vi "Micrometer Heading.vi"() -> ()   [LabVIEW 2024]
uses:
  Library/Class/Renishaw-XL80/Renishaw-XL80.lvclass
  Library/Class/Renishaw-XL80_EMU/Renishaw-XL80_EMU.lvclass
  <vilib>/Utility/file.llb/Write Delimited Spreadsheet (string).vi
panel:
  in  "Nominal":dbl[](array[numeric]) format="%.6f"
  in  "Delete RG":bool
  in  "Delete RB":bool
  out "Signal":dbl(slide) scale=0.0..31.0
  in  "sign_mode":bool
  out "ScanCode 2":i16
  in  "Add DUT":bool
  out "Zero Value":dbl format="%_8f"
  out "Mat Temp":dbl[](array[numeric]) caption="Mat Temp(°C)"
  out "Air Temp":dbl caption="Air Temp(°C)"
  in  "Reset":bool
  in  "Connect":bool
  in  "Zero":bool
  out "Serial Number":string caption="Laser Device ID"
  out "Connected":bool
  in  "Read RB":bool
  in  "R1":dbl[](array[numeric]) format="%.6f"
  in  "Clear RB":bool
  in  "Clear Result":bool
  in  "Export to CSV":bool
  in  "Calculate_Save":bool
  in  "Calculation Result":string[][](table)
  in  "Read RG":bool
  in  "R2":dbl[](array[numeric]) format="%.6f"
  in  "Clear RG":bool
  in  "Precision":u16(ring)=4 items=["0 digit", "1 digit", "2 digits", "3 digits", "4 digits", "5 digits", "6 digits"]
  in  "Unit":u16(ring) caption="mm/inch" items=["mm", "inch"]
  out "Measurement":dbl format="%.6f"
  in  "Description":string
  in  "Mat Exp Coef":dbl format="%_4f"
  in  "Manufacturer":string
  in  "Ref equipment ID":string
  in  "Model No.":string
  in  "S/No. or ID":string
  in  "Job No.":string
  out "uncalibrated":dbl
  out "error out 2":errorcluster
  out "ScanCode":i16
  out "mat_c":dbl
  out "C":dbl format="%.7f"
  out "error out":errorcluster
  in  "error IO":errorcluster
  # "Job Info"
  # "Test Parameters"
  # "DUT Info"
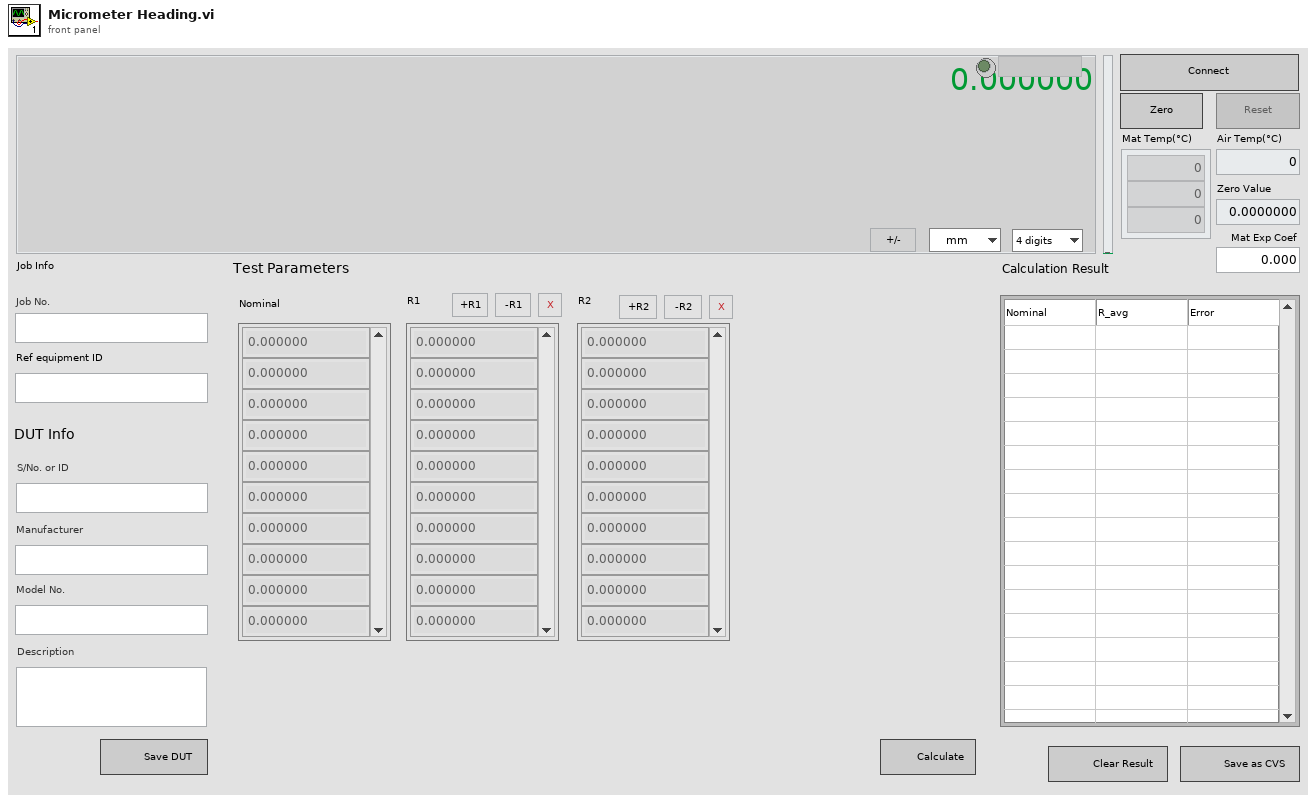
[diagram p1: front panel]
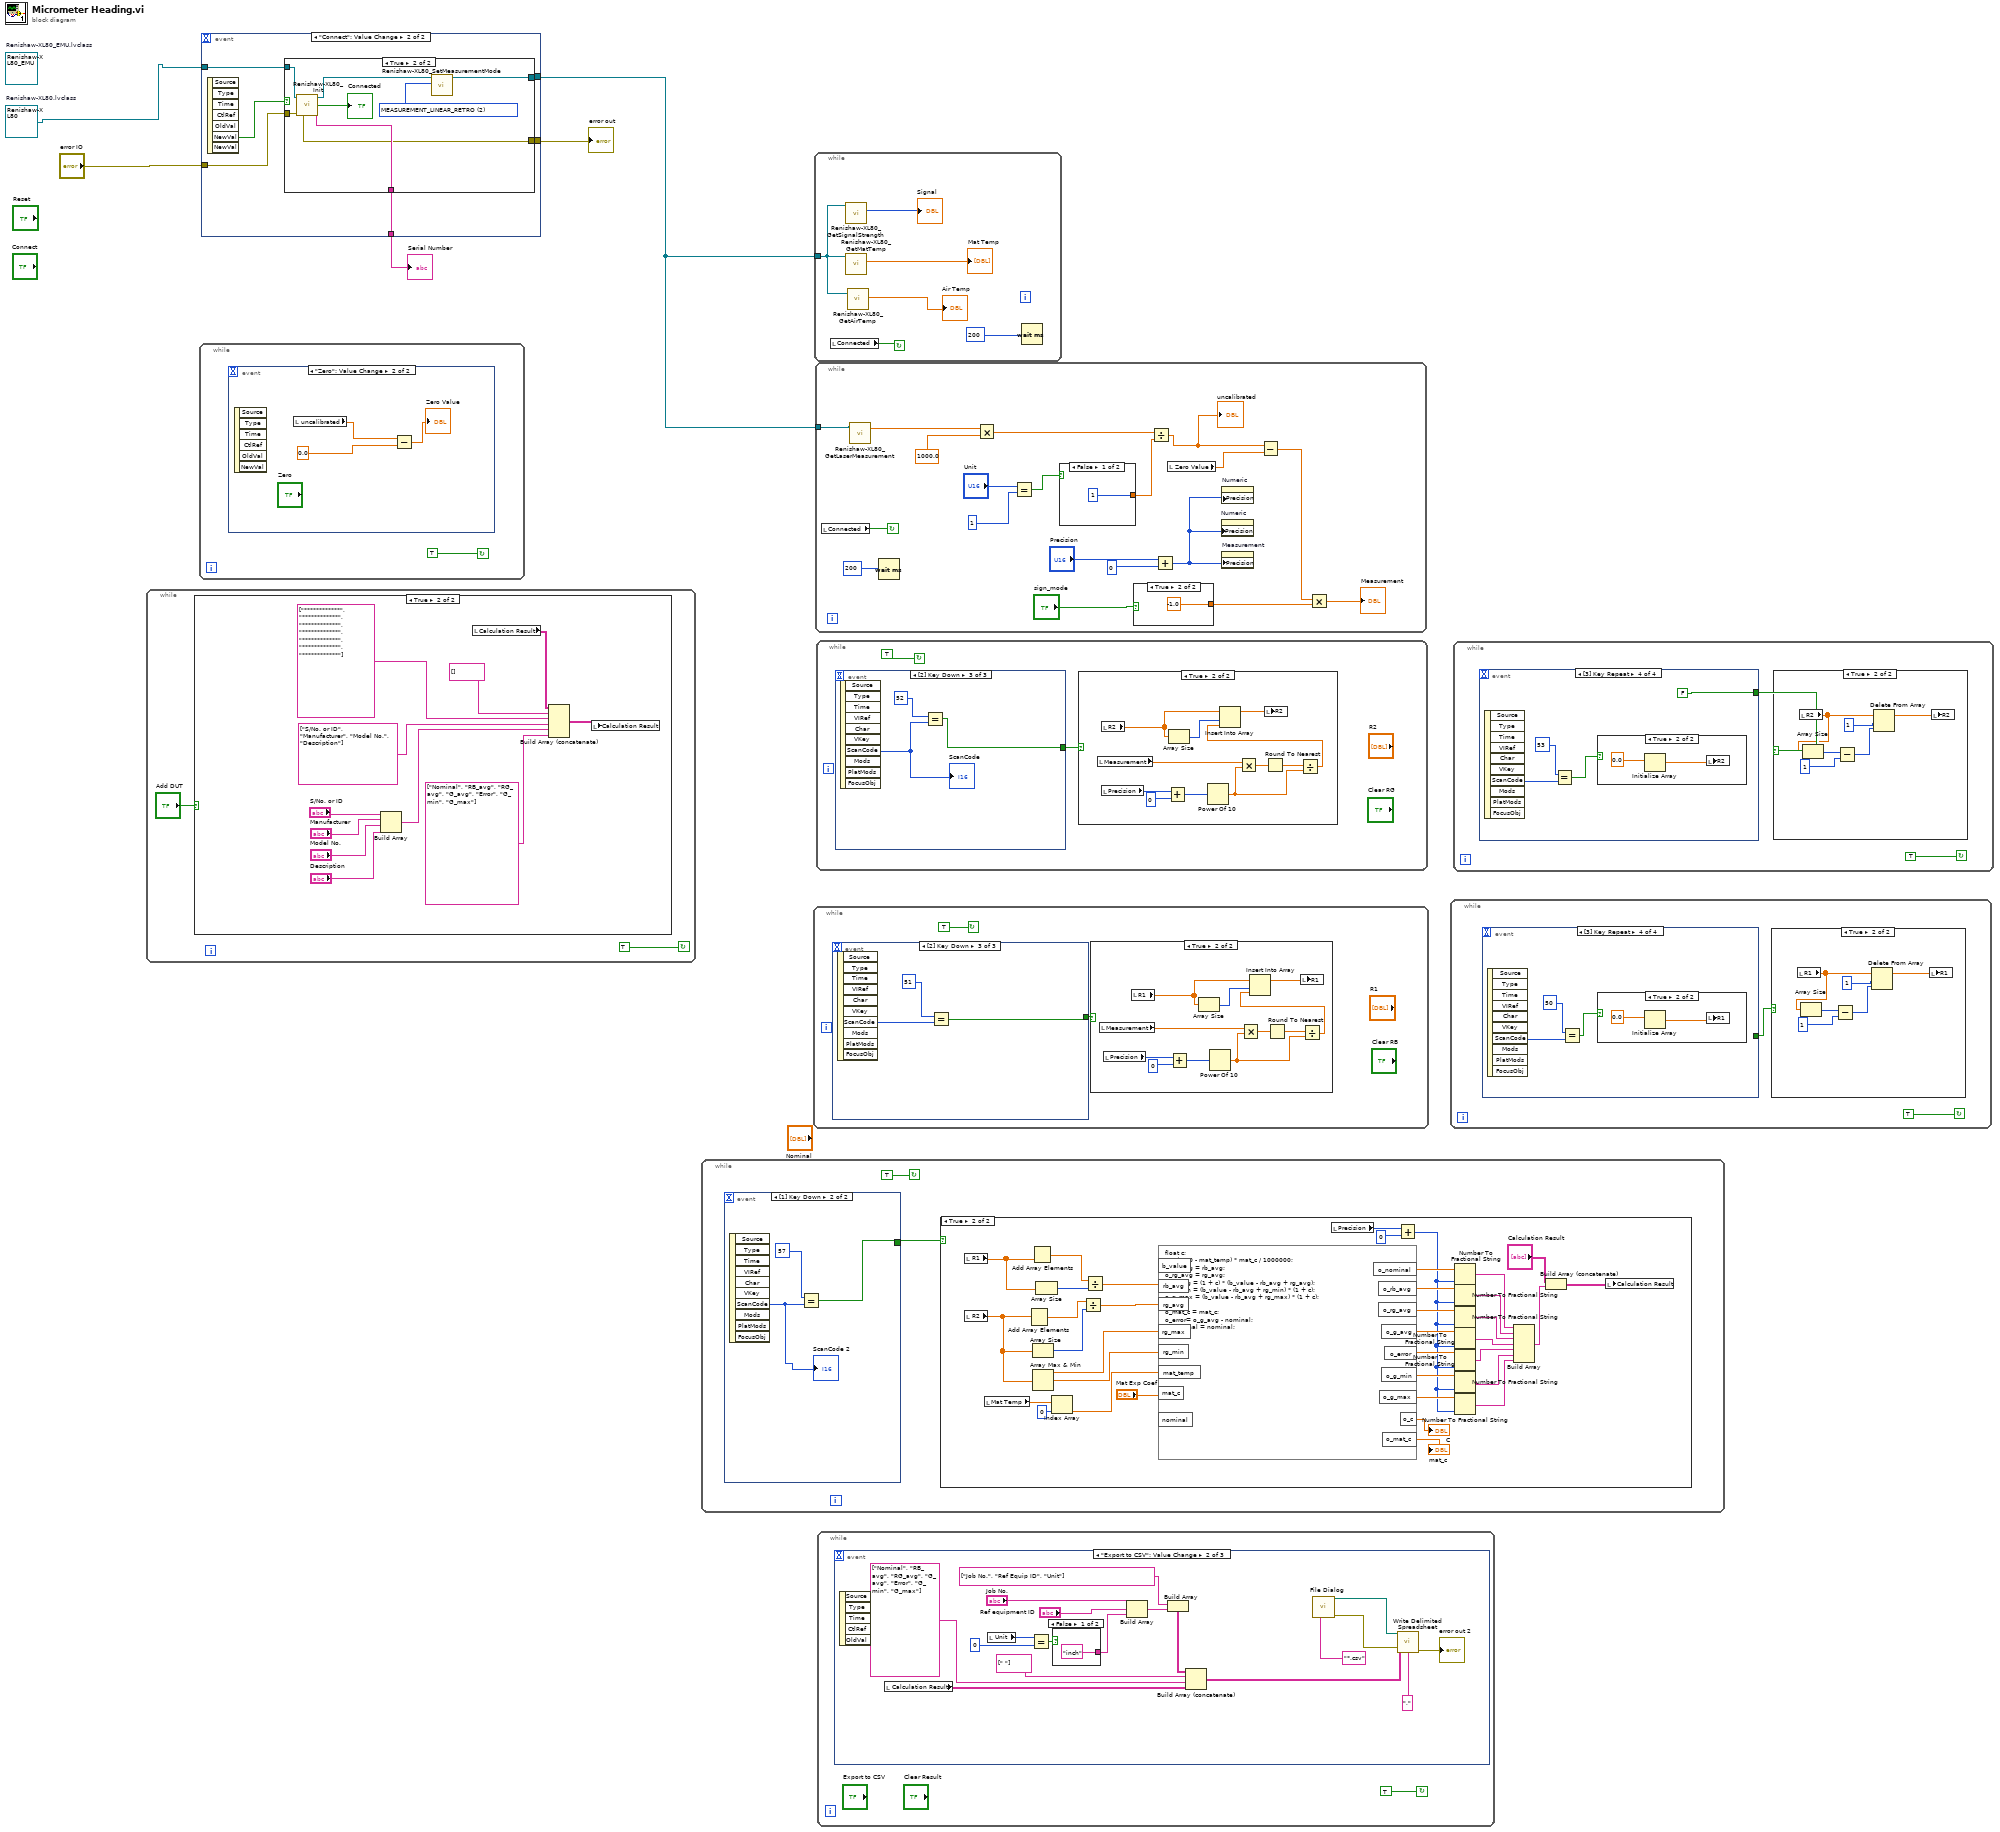
[diagram p0: block diagram]
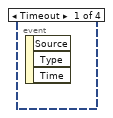
[diagram p3: hidden frame]
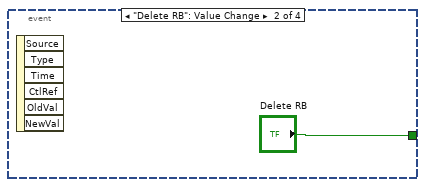
[diagram p4: hidden frame]
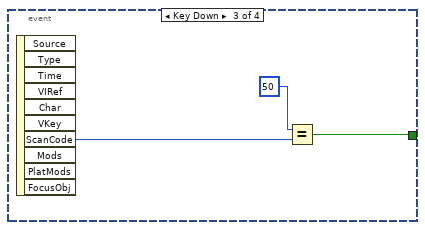
[diagram p5: hidden frame]
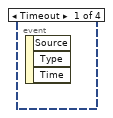
[diagram p8: hidden frame]
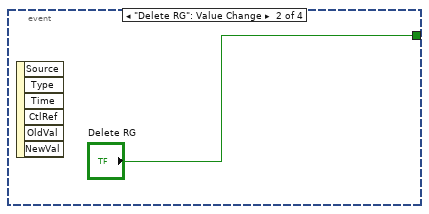
[diagram p9: hidden frame]
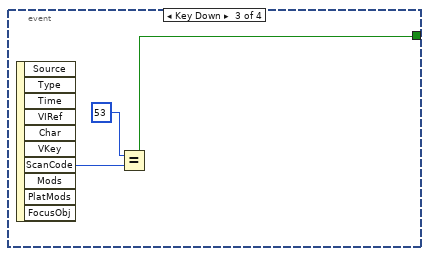
[diagram p10: hidden frame]
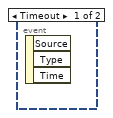
[diagram p13: hidden frame]
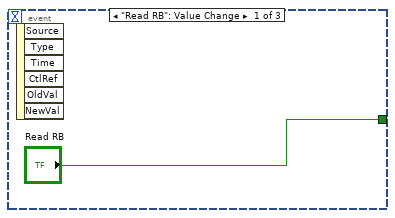
[diagram p15: hidden frame]
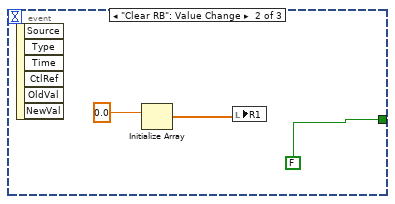
[diagram p16: hidden frame]
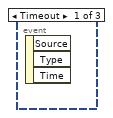
[diagram p17: hidden frame]
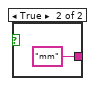
[diagram p18: hidden frame]
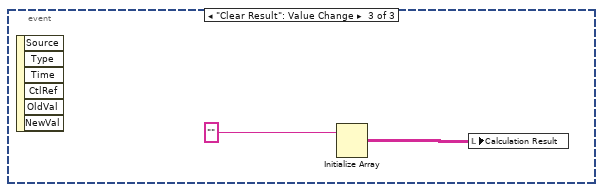
[diagram p19: hidden frame]
diagram:
  (unwired) refnum<class "Renishaw-XL80_EMU.lvclass"> refnum  # Renishaw-XL80_EMU.lvclass
  w1 = refnum<class "Renishaw-XL80.lvclass"> refnum  # Renishaw-XL80.lvclass
  n1 = while {
    stop <- TRUE continue-if-true
    n2 = case shown="True" "Add DUT" {
      frame False {
      }
      frame True {
        n3 = Build Array("S/No. or ID", "Manufacturer", "Model No.", "Description") -> (w10:string[])
        n4 = local read "Calculation Result"() -> (w9:string[][])
        n5 = Build Array (concatenate)(w9, string[] [] ("element"), string[] ["************", "************", "************", "************", "************", "************", "************"], string[] ["S/No. or ID", "Manufacturer", "Model No.", "Description"], w10, string[] ["Nominal", "RB_avg", "RG_avg", "G_avg", "Error", "G_min", "G_max"]) -> (w14:string[][])
        n6 = local write "Calculation Result"(w14) -> ()
      }
    }
  }
  n7 = while {
    stop <- TRUE continue-if-true
    n8 = event shown="[1] \"Zero\": Value Change" {
      selector: _ -> [_ _]
      dyn-events: _ -> [_ _]
      timeout: _ -> [_ _]
      event Timeout {
        n9 = event-data() -> ()  [unwired: 1 in, 3 out]
      }
      event "Zero": Value Change {
        n10 = event-data() -> ()  [unwired: 1 in, 6 out]
        n11 = local read "uncalibrated"() -> (w22:dbl)
        n12 = Subtract(x=w22, y=0.0) -> (x-y=→"Zero Value":dbl)
      }
    }
  }
  n13 = event shown="[1] \"Connect\": Value Change" {
    selector: _ -> [_ _]
    dyn-events: _ -> [_ _]
    timeout: _ -> [_ _]
    tunnel: w1 -> [_ w28]
    tunnel: [_ w27] -> w4
    tunnel: [_ w26] -> w5
    tunnel: "error IO" -> [_ w25]
    tunnel: [_ w24] -> w3
    event Timeout {
      n14 = event-data() -> ()  [unwired: 1 in, 3 out]
    }
    event "Connect": Value Change {
      n15 = event-data() -> ("NewVal"=w23:bool)  [unwired: 1 in, 6 out]
      n16 = case shown="True" w23 {
        tunnel: w28 -> [w33 w41]
        tunnel: ["N/A" ("Serial Number") w40] -> w26
        tunnel: [w32 w35] -> w27
        tunnel: w25 -> [w31 w39]
        tunnel: [w30 w38] -> w24
        frame False {
          n17 = call-dynamic "Renishaw-XL80_Close.vi"("error in (no error)"=w31, "Renishaw-XL80 in"=w33) -> ("error out"=w30:errorcluster, "Renishaw-XL80 out"=w32:refnum<class "Renishaw-XL80.lvclass">)  [unwired: 8 in]
        }
        frame True {
          w34 = 2 items=["MEASUREMENT_INDETERMINATE", "MEASUREMENT_LINEAR_PLANE", "MEASUREMENT_LINEAR_RETRO", "MEASUREMENT_ANGULAR", "MEASUREMENT_STRAIGHTNESS_SHORT", "MEASUREMENT_STRAIGHTNESS_LONG", "MEASUREMENT_VELOCITY_RETRO"] ("MeasurementMode")
          n18 = call-dynamic "Renishaw-XL80_Init.vi"("error in (no error)"=w39, "Renishaw-XL80 in"=w41) -> ("error out"=w38:errorcluster, "Serial Number"=w40:string, "Connect"=→"Connected":bool, "Renishaw-XL80 out"=w36:refnum<class "Renishaw-XL80.lvclass">)  [unwired: 6 in]
          n19 = call-dynamic "Renishaw-XL80_SetMeasurementMode.vi"("MeasurementMode"=w34, "Renishaw-XL80 in"=w36) -> ("Renishaw-XL80 out"=w35:refnum<class "Renishaw-XL80.lvclass">)  [unwired: 8 in, 1 out]
        }
      }
    }
  }
  "error out" <- w3
  "Serial Number" <- w5
  n20 = while {
    stop <- TRUE continue-if-true
    n21 = event shown="[1] Key Down" {
      selector: _ -> [_ _]
      dyn-events: _ -> [_ _]
      timeout: _ -> [_ _]
      tunnel: ["Calculate_Save" w83] -> w42
      event "Calculate_Save": Value Change {
        n22 = event-data() -> ()  [unwired: 1 in, 6 out]
      }
      event Key Down {
        n23 = event-data() -> ("ScanCode"=w84:i16)  [unwired: 1 in, 9 out]
        "ScanCode 2" <- w84
        n24 = Equal?(x=i16 57 ("y"), y=w84) -> (x = y?=w83:bool)
      }
    }
    n25 = case shown="True" w42 {
      frame False {
      }
      frame True {
        n26 = local read "R1"() -> (w81:dbl[])
        n27 = local read "R2"() -> (w70:dbl[])
        n28 = local read "Mat Temp"() -> (w59:dbl[])
        n29 = Add Array Elements(numeric array=w70) -> (sum=w77:dbl)
        n30 = Add Array Elements(numeric array=w81) -> (sum=w80:dbl)
        n31 = Array Size(array=w70) -> (size(s)=w78:i32)
        n32 = Array Max & Min(array=w70) -> (max value=w69:dbl, min value=w68:dbl)  [unwired: 2 out]
        n33 = Array Size(array=w81) -> (size(s)=w79:i32)
        n34 = Index Array(array=w59, index=0) -> (element=w57:dbl)
        n35 = Divide(x=w77, y=w78) -> (x/y=w72:dbl)
        n36 = Divide(x=w80, y=w79) -> (x/y=w73:dbl)
        n37 = formula code="float c;\nc = (20.0 - mat_temp) * mat_c / 1000000;\no_rb_avg = rb_avg;\no_rg_avg = rg_avg;\no_g_avg = (1 + c) * (b_value - rb_avg + rg_avg);\no_g_min = (b_value - rb_avg + rg_min) * (1 + c);\no_g_max = (b_value - rb_avg + rg_max) * (1 + c);\no_c = c;\no_mat_c = mat_c;\no_error= o_g_avg - nominal;\no_nominal = nominal;"("rb_avg"=w73, "rg_avg"=w72, "mat_c"="Mat Exp Coef", "rg_min"=w68, "rg_max"=w69, "mat_temp"=w57) -> ("b_value"=w71:dbl, "o_g_avg"=w64:dbl, "o_g_min"=w63:dbl, "o_g_max"=w62:dbl, "o_rb_avg"=w66:dbl, "o_rg_avg"=w65:dbl, "o_c"=→"C":dbl, "o_mat_c"=→"mat_c":dbl, "o_nominal"=w49:dbl, "o_error"=w53:dbl, "nominal"=w47:dbl)
        n38 = local read "Precision"() -> (w45:u16)
        n39 = Add(x=w45, y=u16 0) -> (x+y=w44:u16)
        n40 = Number To Fractional String(number=w49, precision (6)=w44) -> (F-format string=w48:string)  [unwired: 2 in]
        n41 = Number To Fractional String(number=w66, precision (6)=w44) -> (F-format string=w67:string)  [unwired: 2 in]
        n42 = Number To Fractional String(number=w65, precision (6)=w44) -> (F-format string=w61:string)  [unwired: 2 in]
        n43 = Number To Fractional String(number=w64, precision (6)=w44) -> (F-format string=w60:string)  [unwired: 2 in]
        n44 = Number To Fractional String(number=w53, precision (6)=w44) -> (F-format string=w50:string)  [unwired: 2 in]
        n45 = Number To Fractional String(number=w63, precision (6)=w44) -> (F-format string=w51:string)  [unwired: 2 in]
        n46 = Number To Fractional String(number=w62, precision (6)=w44) -> (F-format string=w52:string)  [unwired: 2 in]
        n47 = Build Array(w48, w67, w61, w60, w50, w51, w52) -> (w75:string[])
        n48 = Build Array (concatenate)("Calculation Result", w75) -> (w76:string[][])
        n49 = local write "Calculation Result"(w76) -> ()
      }
    }
  }
  n50 = while {
    stop <- TRUE continue-if-true
    n51 = event shown="[2] Key Down" {
      selector: _ -> [_ _ _]
      dyn-events: _ -> [_ _ _]
      timeout: _ -> [_ _ _]
      tunnel: ["Read RB" FALSE ("Read RB") w103] -> w87
      event "Read RB": Value Change {
        n52 = event-data() -> ()  [unwired: 1 in, 6 out]
      }
      event "Clear RB": Value Change {
        n53 = event-data() -> ()  [unwired: 1 in, 6 out]
        n54 = Initialize Array(0.0 ("element")) -> (w102:dbl[])  [unwired: 1 in]
        n55 = local write "R1"(w102) -> ()
      }
      event Key Down {
        n56 = event-data() -> ("ScanCode"=w105:i16)  [unwired: 1 in, 9 out]
        n57 = Equal?(x=i16 51 ("y"), y=w105) -> (x = y?=w103:bool)
      }
    }
    n58 = case shown="True" w87 {
      frame False {
      }
      frame True {
        n59 = local read "Measurement"() -> (w91:dbl)
        n60 = local read "Precision"() -> (w90:u16)
        n61 = local read "R1"() -> (w97:dbl[])
        n62 = Add(x=w90, y=u16 0) -> (x+y=w92:u16)
        n63 = Array Size(array=w97) -> (size(s)=w96:i32)
        n64 = Power Of 10(x=w92) -> (10^x=w95:dbl)
        n65 = Multiply(x=w91, y=w95) -> (x*y=w93:dbl)
        n66 = Round To Nearest(number=w93) -> (nearest integer value=w94:dbl)
        n67 = Divide(x=w94, y=w95) -> (x/y=w88:dbl)
        n68 = Insert Into Array(array=w97, index=w96, new element=w88) -> (w98:dbl[])
        n69 = local write "R1"(w98) -> ()
      }
    }
  }
  n70 = while {
    tunnel: w4 -> [w107]
    stop <- w108 continue-if-true
    n71 = local read "Connected"() -> (w108:bool)
    n72 = call-dynamic "Renishaw-XL80_GetSignalStrength.vi"("Renishaw-XL80 in"=w107) -> ("Signal Strength"=→"Signal":i16)  [unwired: 8 in, 2 out]
    n73 = call-dynamic "Renishaw-XL80_GetMatTemp.vi"("Renishaw-XL80 in"=w107) -> ("Temperature Array"=→"Mat Temp":dbl[])  [unwired: 7 in, 3 out]
    n74 = call-dynamic "Renishaw-XL80_GetAirTemp.vi"("Renishaw-XL80 in"=w107) -> ("GetAirTemp"=→"Air Temp":dbl)  [unwired: 7 in, 3 out]
    n75 = Wait (ms)(milliseconds to wait=u32 200) -> ()  [unwired: 1 out]
  }
  n76 = while {
    tunnel: w4 -> [w130]
    stop <- w119 continue-if-true
    n77 = local read "Connected"() -> (w119:bool)
    n78 = call-dynamic "Renishaw-XL80_GetLaserMeasurement.vi"("Renishaw-XL80 in"=w130) -> ("GetLaserMeasurement"=w128:dbl)  [unwired: 7 in, 3 out]
    n79 = Wait (ms)(milliseconds to wait=u32 200) -> ()  [unwired: 1 out]
    n80 = Multiply(x=w128, y=1000.0) -> (x*y=w120:dbl)
    n81 = Equal?(x="Unit", y=u16 1) -> (x = y?=w122:bool)
    n82 = case shown="False" w122 {
      tunnel: [1 25.4] -> w121
      frame False {
      }
      frame True {
      }
    }
    n83 = case shown="True" "sign_mode" {
      tunnel: [1.0 -1.0] -> w114
      frame False {
      }
      frame True {
      }
    }
    n84 = Divide(x=w120, y=w121) -> (x/y=w117:dbl)
    "uncalibrated" <- w117
    n85 = Add(x="Precision", y=u16 0) -> (x+y=w116:u16)
    n86 = local read "Zero Value"() -> (w118:dbl)
    n87 = property on="Numeric" class="DigNum (strict)"("Precision"=w116) -> ()  [unwired: 2 in, 2 out]
    n88 = property on="Numeric" class="DigNum (strict)"("Precision"=w116) -> ()  [unwired: 2 in, 2 out]
    n89 = property on="Measurement" class="DigNum (strict)"("Precision"=w116) -> ()  [unwired: 2 in, 2 out]
    n90 = Subtract(x=w117, y=w118) -> (x-y=w113:dbl)
    n91 = Multiply(x=w113, y=w114) -> (x*y=→"Measurement":dbl)
  }
  n92 = while {
    stop <- TRUE continue-if-true
    n93 = event shown="[2] Key Down" {
      selector: _ -> [_ _ _]
      dyn-events: _ -> [_ _ _]
      timeout: _ -> [_ _ _]
      tunnel: ["Read RG" FALSE ("Read RG") w153] -> w136
      event "Read RG": Value Change {
        n94 = event-data() -> ()  [unwired: 1 in, 6 out]
      }
      event "Clear RG": Value Change {
        n95 = event-data() -> ()  [unwired: 1 in, 6 out]
        n96 = Initialize Array(0.0 ("element")) -> (w150:dbl[])  [unwired: 1 in]
        n97 = local write "R2"(w150) -> ()
      }
      event Key Down {
        n98 = event-data() -> ("ScanCode"=w152:i16)  [unwired: 1 in, 9 out]
        "ScanCode" <- w152
        n99 = Equal?(x=i16 52 ("y"), y=w152) -> (x = y?=w153:bool)
      }
    }
    n100 = case shown="True" w136 {
      frame False {
      }
      frame True {
        n101 = local read "Measurement"() -> (w142:dbl)
        n102 = local read "R2"() -> (w146:dbl[])
        n103 = local read "Precision"() -> (w143:u16)
        n104 = Add(x=w143, y=u16 0) -> (x+y=w141:u16)
        n105 = Array Size(array=w146) -> (size(s)=w145:i32)
        n106 = Power Of 10(x=w141) -> (10^x=w138:dbl)
        n107 = Multiply(x=w142, y=w138) -> (x*y=w140:dbl)
        n108 = Round To Nearest(number=w140) -> (nearest integer value=w139:dbl)
        n109 = Divide(x=w139, y=w138) -> (x/y=w137:dbl)
        n110 = Insert Into Array(array=w146, index=w145, new element=w137) -> (w147:dbl[])
        n111 = local write "R2"(w147) -> ()
      }
    }
  }
  n112 = while {
    stop <- TRUE continue-if-true
    n113 = event shown="[1] \"Export to CSV\": Value Change" {
      selector: _ -> [_ _ _]
      dyn-events: _ -> [_ _ _]
      timeout: _ -> [_ _ _]
      event Timeout {
        n114 = event-data() -> ()  [unwired: 1 in, 3 out]
      }
      event "Export to CSV": Value Change {
        n115 = event-data() -> ()  [unwired: 1 in, 5 out]
        n116 = local read "Calculation Result"() -> (w170:string[][])
        n117 = local read "Unit"() -> (w162:u16)
        n118 = Equal?(x=w162, y=u16 0) -> (x = y?=w160:bool)
        n119 = case shown="False" w160 {
          tunnel: ["inch" "mm"] -> w159
          frame False {
          }
          frame True {
          }
        }
        n120 = Build Array("Job No.", "Ref equipment ID", w159) -> (w157:string[])
        n121 = Build Array(string[] ["Job No.", "Ref Equip ID", "Unit"] ("element"), w157) -> (w156:string[][])
        n122 = Build Array (concatenate)(w156, string[] [" "] ("array"), string[] ["Nominal", "RB_avg", "RG_avg", "G_avg", "Error", "G_min", "G_max"], w170) -> (w172:string[][])
        n123 = call "File Dialog"("pattern (all files)"="*.csv") -> ("selected path"=w169:path, "error out"=w166:errorcluster)  [unwired: 11 in, 2 out]
        n124 = call-poly <vilib>:"Write Delimited Spreadsheet.vi"("file path (dialog if empty)"=w169, "2D data"=w172, "error in (no error)"=w166, "delimiter (\\t)"="," ("delimiter (\\t)")) -> ("error out"=→"error out 2":errorcluster)  [unwired: 10 in, 1 out]
      }
      event "Clear Result": Value Change {
        n125 = event-data() -> ()  [unwired: 1 in, 6 out]
        n126 = Initialize Array("") -> (w177:string[][])  [unwired: 2 in]
        n127 = local write "Calculation Result"(w177) -> ()
      }
    }
  }
  n128 = while {
    stop <- TRUE continue-if-true
    n129 = event shown="[3] Key Repeat" {
      selector: _ -> [_ _ _ _]
      dyn-events: _ -> [_ _ _ _]
      timeout: _ -> [_ _ _ _]
      tunnel: [_ "Delete RB" w187 _] -> w178
      event Timeout {
        n130 = event-data() -> ()  [unwired: 1 in, 3 out]
      }
      event "Delete RB": Value Change {
        n131 = event-data() -> ()  [unwired: 1 in, 6 out]
      }
      event Key Down {
        n132 = event-data() -> ("ScanCode"=w188:i16)  [unwired: 1 in, 9 out]
        n133 = Equal?(x=i16 50 ("y"), y=w188) -> (x = y?=w187:bool)
      }
      event Key Repeat {
        n134 = event-data() -> ("ScanCode"=w191:i16)  [unwired: 1 in, 9 out]
        n135 = Equal?(x=i16 50 ("y"), y=w191) -> (x = y?=w190:bool)
        n136 = case shown="True" w190 {
          frame False {
          }
          frame True {
            n137 = Initialize Array(0.0 ("element")) -> (w194:dbl[])  [unwired: 1 in]
            n138 = local write "R1"(w194) -> ()
          }
        }
      }
    }
    n139 = case shown="True" w178 {
      frame False {
      }
      frame True {
        n140 = local read "R1"() -> (w184:dbl[])
        n141 = Array Size(array=w184) -> (size(s)=w183:i32)
        n142 = Subtract(x=w183, y=1) -> (x-y=w181:i32)
        n143 = Delete From Array(array=w184, length=1, index=w181) -> (array with subset deleted=w180:dbl[])  [unwired: 1 out]
        n144 = local write "R1"(w180) -> ()
      }
    }
  }
  n145 = while {
    stop <- TRUE continue-if-true
    n146 = event shown="[3] Key Repeat" {
      selector: _ -> [_ _ _ _]
      dyn-events: _ -> [_ _ _ _]
      timeout: _ -> [_ _ _ _]
      tunnel: [_ "Delete RG" w204 FALSE ("Delete RG")] -> w195
      event Timeout {
        n147 = event-data() -> ()  [unwired: 1 in, 3 out]
      }
      event "Delete RG": Value Change {
        n148 = event-data() -> ()  [unwired: 1 in, 6 out]
      }
      event Key Down {
        n149 = event-data() -> ("ScanCode"=w205:i16)  [unwired: 1 in, 9 out]
        n150 = Equal?(x=i16 53 ("y"), y=w205) -> (x = y?=w204:bool)
      }
      event Key Repeat {
        n151 = event-data() -> ("ScanCode"=w209:i16)  [unwired: 1 in, 9 out]
        n152 = Equal?(x=i16 53 ("y"), y=w209) -> (x = y?=w207:bool)
        n153 = case shown="True" w207 {
          frame False {
          }
          frame True {
            n154 = Initialize Array(0.0 ("element")) -> (w212:dbl[])  [unwired: 1 in]
            n155 = local write "R2"(w212) -> ()
          }
        }
      }
    }
    n156 = case shown="True" w195 {
      frame False {
      }
      frame True {
        n157 = local read "R2"() -> (w201:dbl[])
        n158 = Array Size(array=w201) -> (size(s)=w200:i32)
        n159 = Subtract(x=w200, y=1) -> (x-y=w198:i32)
        n160 = Delete From Array(array=w201, length=1, index=w198) -> (array with subset deleted=w197:dbl[])  [unwired: 1 out]
        n161 = local write "R2"(w197) -> ()
      }
    }
  }
